vi "Read Frame Data.vi"(0 "Frame data":string[](array[string]), 9 "Label setting":T1={"with label column?"=FALSE, "label column index"=-1}, 11 "error in (no error)":errorcluster) -> (4 "data":dbl[][](array[numeric]), 6 "Hand sign":i32[](array[numeric]), 8 "feature names":string[](array[string]), 15 "error out":errorcluster)   [LabVIEW 2017, in "MachineLearning.lvlib"]
doc: "Reads data and labels from a CSV file. The first row of the CSV file must contain the feature names."
uses:
  MachineLearning.lvlib
  TypeDefs/Label Setting.ctl
  LeapMotion/LeapMotion.lvlib
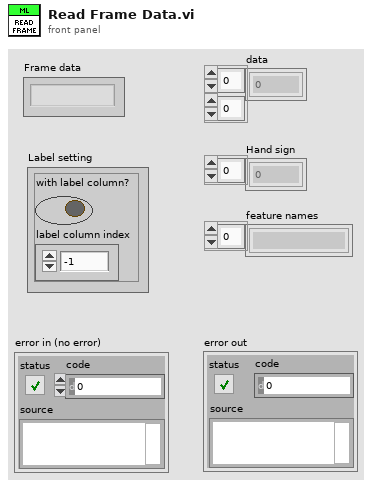
[diagram p1: front panel]
types:
  T1 = typedef "MachineLearning.lvlib/Label Setting.ctl" = cluster{"with label column?":bool, "label column index":i32}
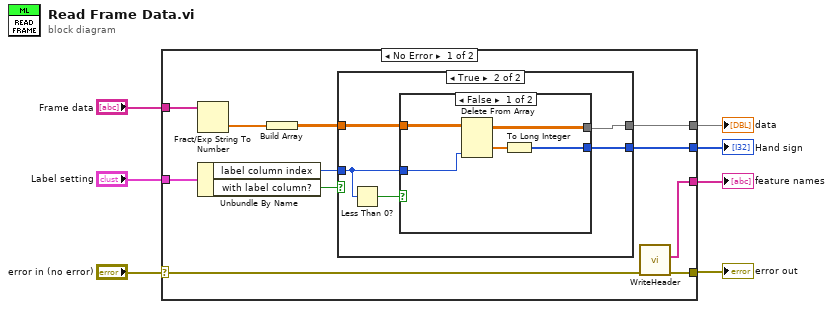
[diagram p0: block diagram]
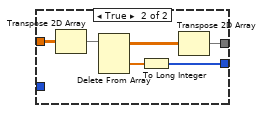
[diagram p3: hidden frame]
diagram:
  n1 = case shown="No Error" "error in (no error)" {
    selector: "error in (no error)" -> [w10 w36]
    tunnel: [w18 _] -> w7
    tunnel: [w17 _] -> w6
    tunnel: [w8 _] -> w4
    tunnel: [w9 w36] -> w3
    tunnel: "Label setting" -> [w16 _]
    tunnel: "Frame data" -> [w13 _]
    frame No Error {
      n2 = Fract/Exp String To Number(string=w13) -> (number=w12:dbl[])  [unwired: 3 in, 1 out]
      n3 = Unbundle By Name(w16) -> ("label column index"=w14:i32, "with label column?"=w15:bool)
      n4 = Build Array(w12) -> (w11:dbl[][])
      n5 = case shown="True" w15 {
        tunnel: [w19 w20] -> w18
        tunnel: [_ w24] -> w17
        tunnel: w14 -> [_ w23]
        tunnel: w11 -> [w19 w21]
        frame False {
        }
        frame True {
          n6 = Less Than 0?(x=w23) -> (x < 0?=w22:bool)
          n7 = case shown="False" w22 {
            tunnel: [w29 w31] -> w20
            tunnel: [w27 w34] -> w24
            tunnel: w23 -> [w26 _]
            tunnel: w21 -> [w25 w30]
            frame False {
              n8 = Delete From Array(array=w25, index (col)=w26) -> (deleted portion=w28:dbl[], array with subset deleted=w29:dbl[][])  [unwired: 2 in]
              n9 = To Long Integer(number=w28) -> (32bit integer=w27:i32[])
            }
            frame True {
              n10 = Transpose 2D Array(2D array=w30) -> (transposed array=w33:dbl[][])
              n11 = Delete From Array(array=w33) -> (deleted portion=w35:dbl[], array with subset deleted=w32:dbl[][])  [unwired: 3 in]
              n12 = To Long Integer(number=w35) -> (32bit integer=w34:i32[])
              n13 = Transpose 2D Array(2D array=w32) -> (transposed array=w31:dbl[][])
            }
          }
        }
      }
      n14 = call "WriteHeader.vi"("Error in"=w10) -> ("Error out"=w9:errorcluster, "Header string array"=w8:string[])  [unwired: 9 in]
    }
    frame Error {
    }
  }
  "data" <- w7
  "feature names" <- w4
  "Hand sign" <- w6
  "error out" <- w3
